vi "Destroy.vi"(8 "error in (no error)":errorcluster, 11 "Name Space in":refnum<class "Name Space.lvclass">) -> (0 "error out":errorcluster)   [LabVIEW 2020, in "Test Executive.lvlib" / "Name Space.lvclass"]
uses:
  <vilib>/gpm_packages/@cs/test-executive/Source/Test Executive/Name Space/Name Space.lvclass
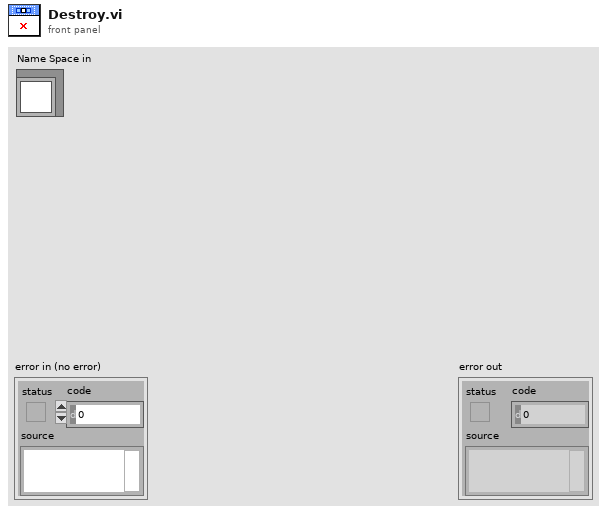
[diagram p1: front panel]
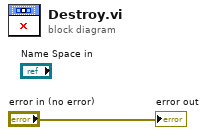
[diagram p0: block diagram]
diagram:
  "error out" <- "error in (no error)"
